vi "Get Dev Product Type.vi"(8 "error in (no error)":errorcluster, 11 "Refnum in":refnum<k21>) -> (0 "error out":errorcluster, 1 "DevIsSimulated":bool, 2 "DAQ Type":T1, 3 "Refnum out":refnum<k21>)   [LabVIEW 2016, in "LockinDAQ.lvclass"]
uses:
  LockinDAQ.lvclass
  Typedefs/DAQType-enum.ctl
  <resource>/objmgr/daqmx.rc
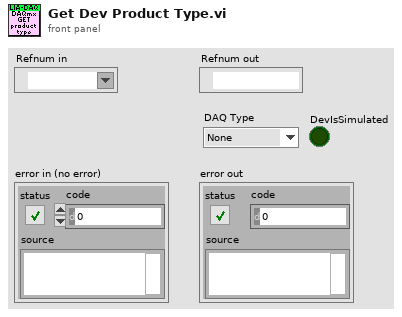
[diagram p1: front panel]
types:
  T1 = typedef "LockinDAQ.lvclass/DAQType-enum.ctl" = enum16{"None", "USB 4431", "PXI 446x"}
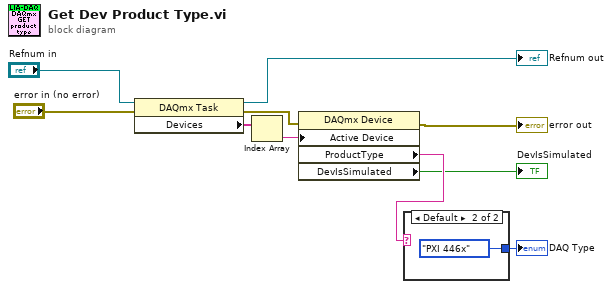
[diagram p0: block diagram]
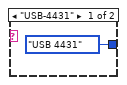
[diagram p2: hidden frame]
diagram:
  n1 = property class="DAQmx Task"(reference="Refnum in", error in="error in (no error)") -> (reference out=→"Refnum out":refnum<k21>, error out=w9:errorcluster, "Devices"=w7:tag[])
  n2 = Index Array(array=w7) -> (element=w4:tag)  [unwired: 1 in]
  n3 = property class="DAQmx Device"(error in=w9, "Active Device"=w4) -> (error out=→"error out":errorcluster, "ProductType"=w3:string, "DevIsSimulated"=→"DevIsSimulated":bool)  [unwired: 1 in, 1 out]
  n4 = case shown="Default" w3 {
    tunnel: [DAQType-enum."USB 4431" ("DAQ Type") DAQType-enum."PXI 446x" ("DAQ Type")] -> w2
    frame "USB-4431" {
    }
    frame Default {
    }
  }
  "DAQ Type" <- w2
